vi "arraycomparelong.vi"(8 "ABS?":bool, 9 "limit type":enum16{"上限", "下限"}(ring), 10 "spec":i32[](array[numeric]), 11 "data":i32[](array[numeric])) -> (3 "result":bool[](array[boolean]))   [LabVIEW 2011]
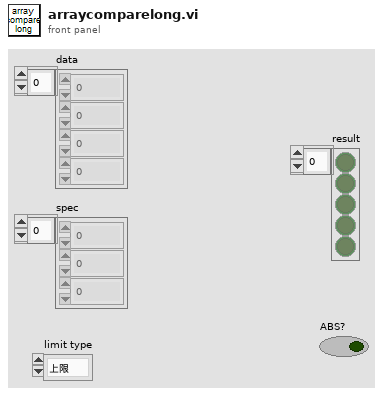
[diagram p1: front panel]
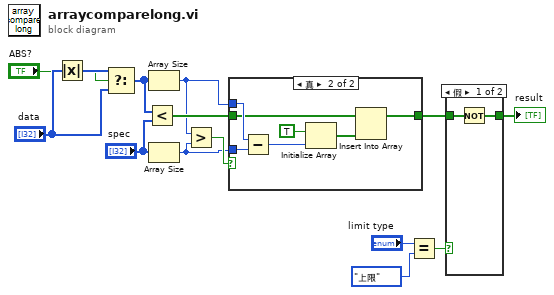
[diagram p0: block diagram]
diagram:
  n1 = Absolute Value(x="data") -> (abs(x)=w3:i32[])
  n2 = Select(t=w3, s="ABS?", f="data") -> (s? t:f=w4:i32[])
  n3 = Less?(x=w4, y="spec") -> (x < y?=w12:bool[])
  n4 = Array Size(array=w4) -> (size(s)=w11:i32)
  n5 = Array Size(array="spec") -> (size(s)=w10:i32)
  n6 = Greater?(x=w11, y=w10) -> (0:w14:bool)
  n7 = case shown="真" w14 {
    tunnel: w12 -> [w15 w18]
    tunnel: [w15 w16] -> w6
    tunnel: w11 -> [_ w22]
    tunnel: w10 -> [_ w21]
    frame False {
    }
    frame True {
      n8 = Subtract(x=w22, y=w21) -> (x-y=w20:i32)
      n9 = Initialize Array(TRUE, w20) -> (w17:bool[])
      n10 = Insert Into Array(array=w18, new element=w17) -> (w16:bool[])  [unwired: 1 in]
    }
  }
  n11 = Equal?(x="limit type", y=enum16{"上限", "下限"}."上限") -> (x = y?=w7:bool)
  n12 = case shown="假" w7 {
    tunnel: w6 -> [w24 w25]
    tunnel: [w23 w25] -> w5
    frame False {
      n13 = Not(x=w24) -> (.not. x?=w23:bool[])
    }
    frame True {
    }
  }
  "result" <- w5
